vi "camera_load.vi"(6 "error in (no error)":errorcluster, 9 "path":path) -> (0 "error out":errorcluster, 1 "serials":u64[](array[numeric]) format="%.0x", 2 "sdks":string[](array[string]), 3 "names":string[](array[string]), 4 "ports":string[](array[string]), 5 "hdf":path)   [LabVIEW 2010]
uses:
  <vilib>/addons/h5labview2/dataset/H5Dread.llb/H5Dread.xnode
  <vilib>/addons/h5labview2/attrib/H5Aread.llb/H5Aread.xnode
  <vilib>/addons/h5labview2/base/H5Equery.vi
  <vilib>/addons/h5labview2/file/H5F.lvlib
  <vilib>/addons/h5labview2/group/H5G.lvlib
  <vilib>/addons/h5labview2/h5labview.lib
panel:
  out "name":string
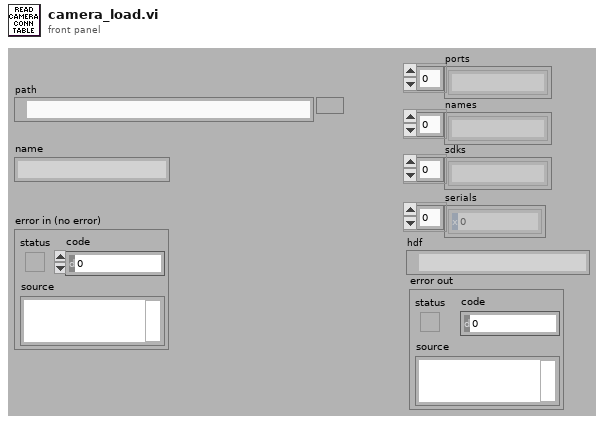
[diagram p1: front panel]
types:
  T1 = typedef "hid_t.ctl" = i32
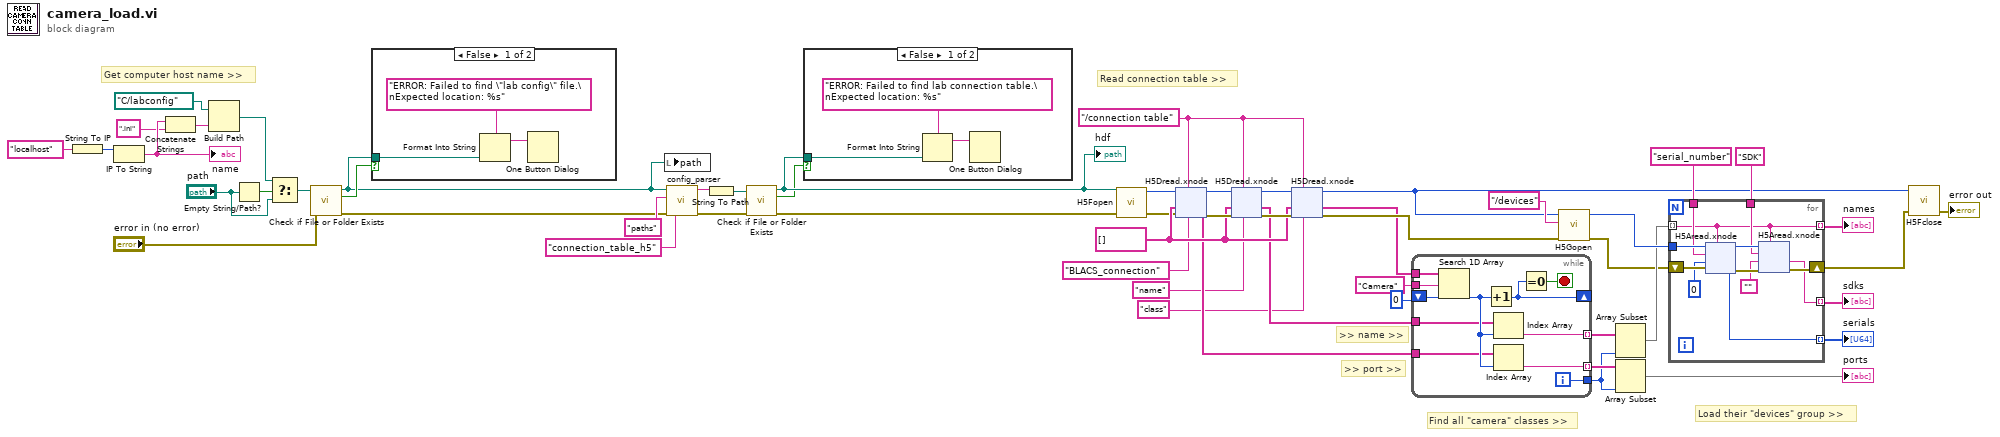
[diagram p0: block diagram]
diagram:
  w10 = string[] []
  w12 = "/connection table" ("table")
  # "Load their \"devices\" group >>"
  # "Find all \"camera\" classes >>"
  # "Read connection table >>"
  # "Get computer host name >>"
  # ">> name >>"
  # ">> port >>"
  n1 = String To IP(1:"localhost" ("name")) -> (0:w35:u32)
  n2 = IP To String(2:w35) -> (0:w33:string)  [unwired: 1 in]
  "name" <- w33
  n3 = Concatenate Strings(w33, ".ini" ("string")) -> (w31:string)
  n4 = Build Path(base path=path "C:/labconfig", name or relative path=w31) -> (appended path=w29:path)
  n5 = Empty String/Path?(string/path="path") -> (empty?=w28:bool)
  n6 = Select(t=w29, s=w28, f="path") -> (s? t:f=w26:path)
  n7 = call <vilib>:"Check if File or Folder Exists.vi"("error in (no error)"="error in (no error)", "path"=w26) -> ("error out"=w25:errorcluster, "file or folder exists?"=w24:bool, "dup path"=w23:path)  [unwired: 7 in]
  n8 = case shown="False" w24 {
    tunnel: w23 -> [w56 _]
    frame False {
      n9 = Format Into String(format string="ERROR: Failed to find \"lab config\" file.\nExpected location: %s", w56) -> (resulting string=w55:string)  [unwired: 2 in, 1 out]
      n10 = One Button Dialog(message=w55) -> ()  [unwired: 1 in, 1 out]
    }
    frame True {
    }
  }
  n11 = local write "path"(w23) -> ()
  n12 = call <userlib>:"config_parser.vi"("error in"=w25, "key"="connection_table_h5", "section"="paths", "path"=w23) -> ("error out"=w21:errorcluster, "result"=w52:string)  [unwired: 2 in]
  n13 = String To Path(string=w52) -> (path=w22:path)
  n14 = call <vilib>:"Check if File or Folder Exists.vi"("error in (no error)"=w21, "path"=w22) -> ("file or folder exists?"=w19:bool, "dup path"=w20:path)  [unwired: 7 in, 1 out]
  "hdf" <- w20
  n15 = case shown="False" w19 {
    tunnel: w20 -> [w59 _]
    frame False {
      n16 = Format Into String(format string="ERROR: Failed to find lab connection table.\nExpected location: %s", w59) -> (resulting string=w58:string)  [unwired: 2 in, 1 out]
      n17 = One Button Dialog(message=w58) -> ()  [unwired: 1 in, 1 out]
    }
    frame True {
    }
  }
  n18 = call <vilib>:"H5Fopen.vi"("error in (no error)"=w21, "path"=w20) -> ("error out"=w5:errorcluster, "ref out"=w4:T1)  [unwired: 2 in]
  n19 = xnode "H5Dread.xnode"("type name (default)"="BLACS_connection", "dataset name (this)"=w12, "error in (no error)"=w5, "default"=w10, "ref in"=w4) -> ("error out"=w11:errorcluster, "data"=w6:string[], "ref out"=w13:i32)  [unwired: 1 in, 1 out]
  n20 = xnode "H5Dread.xnode"("type name (default)"="name", "dataset name (this)"=w12, "error in (no error)"=w11, "default"=w10, "ref in"=w13) -> ("error out"=w16:errorcluster, "data"=w7:string[], "ref out"=w15:i32)  [unwired: 1 in, 1 out]
  n21 = xnode "H5Dread.xnode"("type name (default)"="class", "dataset name (this)"=w12, "error in (no error)"=w16, "default"=w10, "ref in"=w15) -> ("error out"=w9:errorcluster, "data"=w8:string[], "ref out"=w14:i32)  [unwired: 1 in, 1 out]
  n22 = while {
    tunnel: w8 -> [w71]
    tunnel: "Camera" ("element") -> [w70]
    shift-right: [w67] -> _
    shift-left: 0 ("index of element") -> [w69]
    tunnel: w7 -> [w65]
    tunnel: w6 -> [w64]
    tunnel: [w63] -> w47 mode=indexing
    tunnel: [w62] -> w46 mode=indexing
    tunnel: [w61] -> w45
    i -> [w61]
    stop <- w68 stop-if-true
    n23 = Search 1D Array(1D array=w71, element=w70, start index (0)=w69) -> (index of element=w66:i32)
    n24 = Increment(x=w66) -> (x+1=w67:i32)
    n25 = Index Array(array=w65, index=w66) -> (element=w63:string)
    n26 = Index Array(array=w64, index=w66) -> (element=w62:string)
    n27 = Equal To 0?(x=w67) -> (x = 0?=w68:bool)
  }
  n28 = call <vilib>:"H5Gopen.vi"("error in (no error)"=w9, "name"="/devices", "ref in"=w14) -> ("error out"=w37:errorcluster, "group out"=w51:T1)  [unwired: 4 in]
  n29 = Array Subset(array=w47, length=w45) -> (w44:string[])  [unwired: 1 in]
  n30 = Array Subset(array=w46, length=w45) -> (→"ports":string[])  [unwired: 1 in]
  n31 = for {
    tunnel: w51 -> [w83]
    tunnel: w44 -> [w72] mode=indexing
    tunnel: "serial_number" ("attrib_name") -> [w80]
    tunnel: "SDK" ("attrib_name") -> [w75]
    tunnel: [w72] -> w40 mode=indexing
    tunnel: [w73] -> w39 mode=indexing
    tunnel: [w81] -> w38 mode=indexing
    shift-right: [w78] -> w17
    shift-left: w37 -> [w82]
    n32 = xnode "H5Aread.xnode"("object name"=w72, "error in (no error)"=w82, "default"=u64 0, "attrib name"=w80, "ref in"=w83) -> ("error out"=w76:errorcluster, "data"=w81:u64, "ref out"=w77:i32)  [unwired: 1 in, 1 out]
    n33 = xnode "H5Aread.xnode"("object name"=w72, "error in (no error)"=w76, "default"="", "attrib name"=w75, "ref in"=w77) -> ("error out"=w78:errorcluster, "data"=w73:string)  [unwired: 1 in, 2 out]
  }
  "names" <- w40
  "sdks" <- w39
  "serials" <- w38
  n34 = call <vilib>:"H5Fclose.vi"("error in (no error)"=w17, "ref"=w14) -> ("error out"=→"error out":errorcluster)  [unwired: 3 in]
